vi "LinxSpiWriteRead.vi"(5 "CS Configuration":T1, 7 "SPI Channel":u8, 8 "Error In":errorcluster, 9 "SPI Frame Size (0)":u8, 10 "Data":u8[](array[numeric]), 11 "LINX Resource":T3) -> (0 "Error Out":errorcluster, 2 "Data":u8[](array[numeric]), 3 "LINX Resource":T3, 4 "status":i32)   [LabVIEW 2020, in "LMH-LINX.lvlib" / "Local IO.lvlib"]
uses:
  Local IO.lvlib
  Type Defs/LINX Ref.ctl
  Type Defs/Platform.ctl
  Type Defs/Interface.ctl
  Device/Type Defs/LINX Device Config.ctl
  Device/Type Defs/TCP Config.ctl
  Device/Type Defs/Channels.ctl
  Public/Peripherals/SPI/SPI CS Config.ctl
  Type Defs/Peripherals/SPI/SPI CS Logic Level.ctl
  Type Defs/Error Type.ctl
  LMH-LINX.lvlib
  <vilib>/MakerHub/LINX/Resources/liblinxdevice.dll
  Device/Device.lvlib
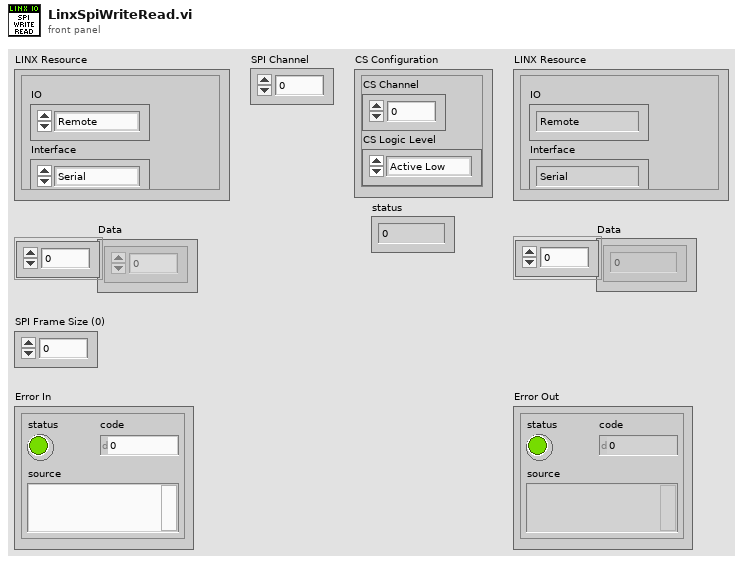
[diagram p1: front panel]
types:
  T1 = typedef "LMH-LINX.lvlib/SPI CS Config.ctl" = cluster{"CS Channel":u8, "CS Logic Level":T2}
  T2 = typedef "LMH-LINX.lvlib/SPI CS Logic Level.ctl" = enum8{"Active Low", "Active High"}
  T3 = typedef "LMH-LINX.lvlib/LINX Ref.ctl" = cluster{"IO":T4, "Interface":T5, "LINX Device Config":T6}
  T4 = typedef "LMH-LINX.lvlib/Platform.ctl" = enum16{"Remote", "Local"}
  T5 = typedef "LMH-LINX.lvlib/Interface.ctl" = enum16{"Serial", "TCP"}
  T6 = typedef "LMH-LINX.lvlib/Device.lvlib/LINX Device Config.ctl" = cluster{"Interface":T5, "COM Port":refnum<visa-resource-name>, "TCP Configuration":T7, "Device Family":u8, "Device ID":u8, "Device Name":string, "TCP Ref":refnum<k5>, "Channels":T8}
  T7 = typedef "LMH-LINX.lvlib/Device.lvlib/TCP Config.ctl" = cluster{"IP Address":string, "Port":u16}
  T8 = typedef "LMH-LINX.lvlib/Channels.ctl" = cluster{"DI":u8[], "DO":u8[], "AI":u8[], "AO":u8[], "PWM":u8[], "QE":u8[], "UART":u8[], "I2C 2":u8[], "SPI":u8[], "CAN":u8[], "Servo":u8[], "AI Ref (V)":dbl, "AI Resolution (Bits)":u8, "AO Ref (V)":dbl, "AO Resolution (Bits)":u8}
  T9 = typedef "LMH-LINX.lvlib/Error Type.ctl" = enum16{"Unknown", "Timeout", "Corrupt Return Packet", "Unable To Connect", "Command Not Supported", "Channel DNE", "Invalid COM Config", "Firmware Version Mismatch", "myRIO Support", "CMD Specific Error", "Local IO Not Supported"}
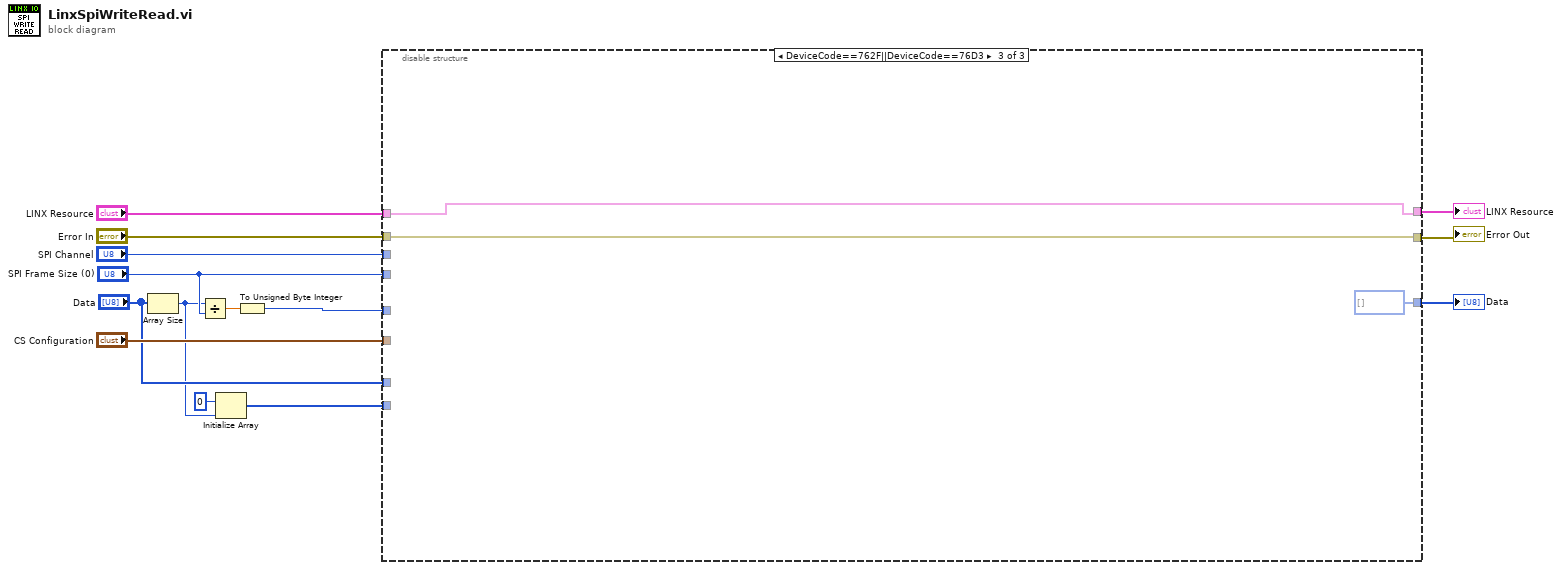
[diagram p0: block diagram]
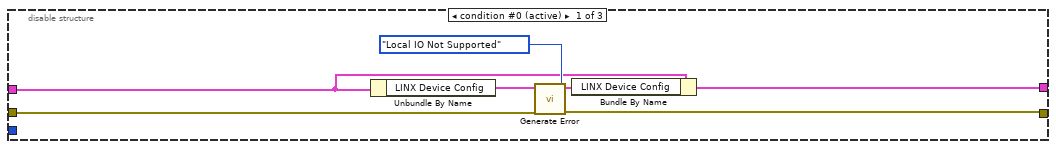
[diagram p2: hidden frame]
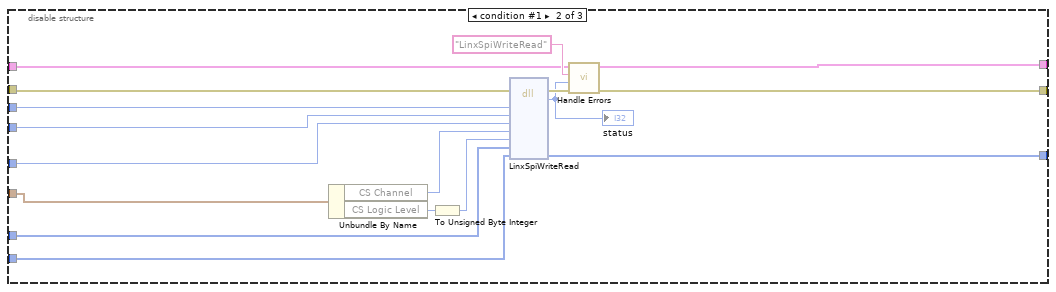
[diagram p3: hidden frame]
diagram:
  n1 = Array Size(array="Data") -> (size(s)=w4:i32)
  n2 = Divide(x=w4, y="SPI Frame Size (0)") -> (x/y=w7:dbl)
  n3 = Initialize Array(u8 0 ("element"), w4) -> (w2:u8[])
  n4 = To Unsigned Byte Integer(number=w7) -> (unsigned 8bit integer=w6:u8)
  n5 = disable-structure shown="DeviceCode==762F||DeviceCode==76D3" {
    disable-tunnel: [w16 w23 w40] -> w14
    disable-tunnel: "LINX Resource" -> [w18 w33 w40]
    disable-tunnel: "Error In" -> [w20 w36 w41]
    disable-tunnel: "SPI Channel" -> [_ w34 _]
    disable-tunnel: [w15 w24 w41] -> w10
    disable-tunnel: "SPI Frame Size (0)" -> [_ w32 _]
    disable-tunnel: w6 -> [_ w30 _]
    disable-tunnel: "CS Configuration" -> [_ w31 _]
    disable-tunnel: "Data" -> [_ w26 _]
    disable-tunnel: w2 -> [_ w25 _]
    disable-tunnel: [_ w22 u8[] [] ("Data")] -> w1
    frame condition #0 (active) {
      n6 = Unbundle By Name(w18) -> ("LINX Device Config"=w19:T6)
      n7 = call "Generate Error.vi"("Error In"=w20, "Error Type"=Error_Type."Local IO Not Supported", "LINX Device Config"=w19) -> ("Error Out"=w15:errorcluster, "Dup LINX Device Config"=w17:T6)  [unwired: 7 in]
      n8 = Bundle By Name(cluster=w18, "LINX Device Config"=w17) -> (w16:T3)
    }
    frame condition #1 {
      n9 = Unbundle By Name(w31) -> ("CS Channel"=w29:u8, "CS Logic Level"=w28:T2)
      n10 = To Unsigned Byte Integer(number=w28) -> (unsigned 8bit integer=w27:u8)
      n11 = dll-call lib="C:/Program Files (x86)/National Instruments/LabVIEW 2020/vi.lib/MakerHub/LINX/Resources/liblinxdevice.*" fn="LinxSpiWriteRead"(error in=w36, "channel"=w34, "frameSize"=w32, "numFrames"=w30, "csChan"=w29, "csLL"=w27, "sendBuffer"=w26, "recBuffer"=w25) -> (error out=w37:errorcluster, "status"=w35:i32, "recBuffer"=w22:u8[])  [unwired: 8 in, 1 out]
      "status" <- w35
      n12 = call <vilib>:"Handle Errors.vi"("Error In"=w37, "LinxStatus"=w35, "Function Name"="LinxSpiWriteRead", "LINX Resource"=w33) -> ("Error Out"=w24:errorcluster, "LINX Resource"=w23:T3)  [unwired: 6 in]
    }
    frame condition #2 {
    }
  }
  "LINX Resource" <- w14
  "Error Out" <- w10
  "Data" <- w1
